vi "测试字符串分离.vi"() -> ()   [LabVIEW 2019]
panel:
  out "数字 2":dbl
  out "数字":dbl
  out "字符串":string
  out "数组":string[](array[string])
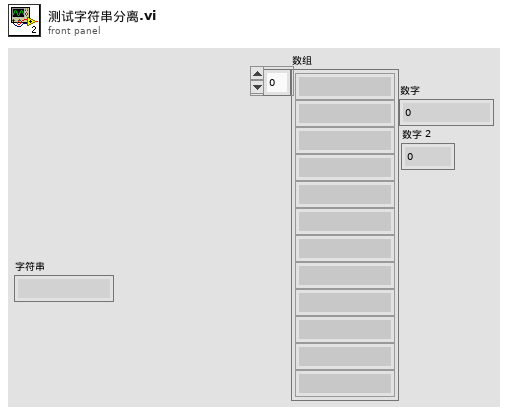
[diagram p1: front panel]
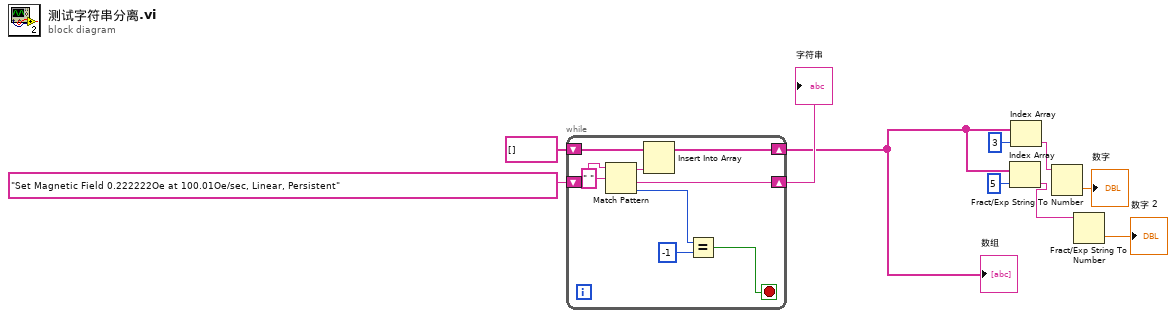
[diagram p0: block diagram]
diagram:
  n1 = while {
    shift-right: [w15] -> w5
    shift-left: string[] [] -> [w14]
    shift-right: [w17] -> w8
    shift-left: "Set Magnetic Field 0.222222Oe at 100.01Oe/sec, Linear, Persistent" -> [w19]
    stop <- w11 stop-if-true
    n2 = Match Pattern(string=w19, regular expression=" " ("正则表达式")) -> (before substring=w16:string, after substring=w17:string, offset past match=w13:i32)  [unwired: 1 in, 1 out]
    n3 = Insert Into Array(array=w14, new element=w16) -> (w15:string[])  [unwired: 1 in]
    n4 = Equal?(x=w13, y=-1) -> (x = y?=w11:bool)
  }
  "数组" <- w5
  "字符串" <- w8
  n5 = Index Array(array=w5, index=5 ("索引")) -> (element=w2:string)
  n6 = Index Array(array=w5, index=3 ("索引")) -> (element=w7:string)
  n7 = Fract/Exp String To Number(string=w7) -> (number=→"数字":dbl)  [unwired: 3 in, 1 out]
  n8 = Fract/Exp String To Number(string=w2) -> (number=→"数字 2":dbl)  [unwired: 3 in, 1 out]
